vi "Alarma_Modulacion_Voltaje_G2.vi"(6 "# iteration":i32, 7 "ID_EQUIPO":i32, 9 "V3_V1":sgl, 10 "V2_V3":sgl, 11 "V1_V2":sgl) -> (3 "Alarma_Mod_Volt out":T1)   [LabVIEW 2018]
panel:
  out "error out":errorcluster
  in  "error in (no error)":errorcluster
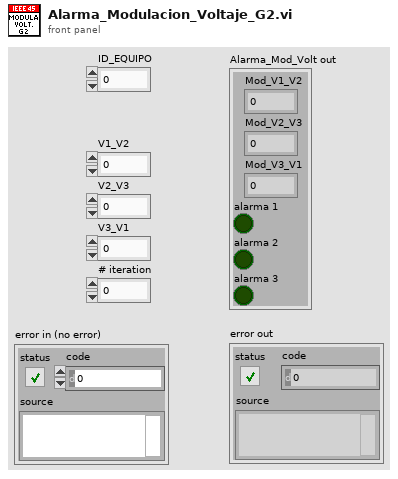
[diagram p1: front panel]
types:
  T1 = cluster{"Mod_V1_V2":sgl, "Mod_V2_V3":sgl, "Mod_V3_V1":sgl, "alarma 1":bool, "alarma 2":bool, "alarma 3":bool}
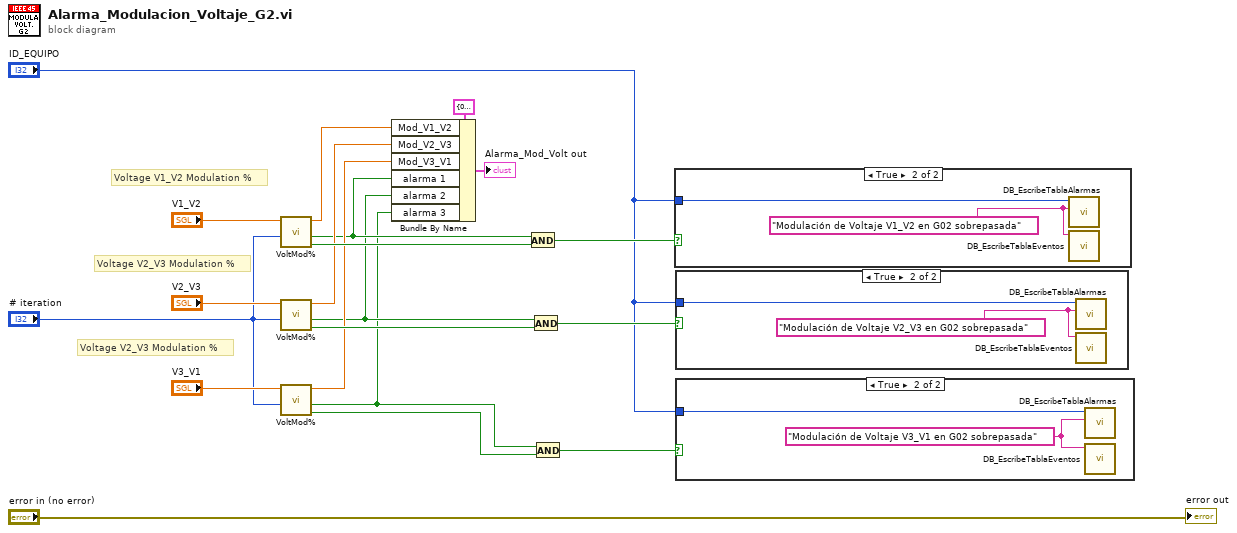
[diagram p0: block diagram]
diagram:
  # "Voltage V2_V3 Modulation %"
  # "Voltage V2_V3 Modulation %"
  # "Voltage V1_V2 Modulation %"
  n1 = call "VoltMod%.vi"("iteracion"="# iteration", "Volt Input"="V1_V2") -> ("cada 10 seg"=w16:bool, "alarma"=w5:bool, "Voltage Modulation (%)"=w8:sgl)  [unwired: 7 in]
  n2 = call "VoltMod%.vi"("iteracion"="# iteration", "Volt Input"="V2_V3") -> ("cada 10 seg"=w14:bool, "alarma"=w4:bool, "Voltage Modulation (%)"=w7:sgl)  [unwired: 7 in]
  n3 = call "VoltMod%.vi"("iteracion"="# iteration", "Volt Input"="V3_V1") -> ("cada 10 seg"=w12:bool, "alarma"=w3:bool, "Voltage Modulation (%)"=w6:sgl)  [unwired: 7 in]
  n4 = Bundle By Name(cluster=T1 {"Mod_V1_V2"=0.0, "Mod_V2_V3"=0.0, "Mod_V3_V1"=0.0, "alarma 1"=FALSE, "alarma 2"=FALSE, "alarma 3"=FALSE} ("Cluster_Mod_Voltaje"), "Mod_V1_V2"=w8, "Mod_V2_V3"=w7, "Mod_V3_V1"=w6, "alarma 1"=w5, "alarma 2"=w4, "alarma 3"=w3) -> (→"Alarma_Mod_Volt out":T1)
  n5 = And(x=w5, y=w16) -> (x .and. y?=w15:bool)
  n6 = And(x=w4, y=w14) -> (x .and. y?=w13:bool)
  n7 = And(x=w3, y=w12) -> (x .and. y?=w11:bool)
  n8 = case shown="True" w15 {
    tunnel: "ID_EQUIPO" -> [_ w22]
    frame False {
    }
    frame True {
      w21 = "Modulación de Voltaje V1_V2 en G02 sobrepasada" ("MOTIVO")
      n9 = call "DB_EscribeTablaAlarmas.vi"("MOTIVO"=w21, "ID_EQUIPO"=w22) -> ()  [unwired: 9 in, 1 out]
      n10 = call "DB_EscribeTablaEventos.vi"("DESCRIPCION"=w21) -> ()  [unwired: 10 in, 1 out]
    }
  }
  n11 = case shown="True" w13 {
    tunnel: "ID_EQUIPO" -> [_ w24]
    frame False {
    }
    frame True {
      w23 = "Modulación de Voltaje V2_V3 en G02 sobrepasada" ("MOTIVO")
      n12 = call "DB_EscribeTablaAlarmas.vi"("MOTIVO"=w23, "ID_EQUIPO"=w24) -> ()  [unwired: 9 in, 1 out]
      n13 = call "DB_EscribeTablaEventos.vi"("DESCRIPCION"=w23) -> ()  [unwired: 10 in, 1 out]
    }
  }
  n14 = case shown="True" w11 {
    tunnel: "ID_EQUIPO" -> [_ w26]
    frame False {
    }
    frame True {
      w25 = "Modulación de Voltaje V3_V1 en G02 sobrepasada" ("MOTIVO")
      n15 = call "DB_EscribeTablaAlarmas.vi"("MOTIVO"=w25, "ID_EQUIPO"=w26) -> ()  [unwired: 9 in, 1 out]
      n16 = call "DB_EscribeTablaEventos.vi"("DESCRIPCION"=w25) -> ()  [unwired: 10 in, 1 out]
    }
  }
  "error out" <- "error in (no error)"
